vi "VisualizePXI_MultiTrig.vi"() -> ()   [LabVIEW 2018, in "Visualization.lvlib" / "VisualizeSync.lvclass"]
doc: "This VI listens for any measurement data associated with the provided PluginName and displays it to the user for analysis. The display is only suitable for data coming from the RoomAlert Plugin."
uses:
  VisualizeSync.lvclass
  <vilib>/event_ctls.llb/usereventprio.ctl
  VisualizeBase/VisualizeBase_class/Requests/clUserEventType.ctl
  <extravilib>/ChannelInstances/Tag-bool/Write With Abort.vi
  <extravilib>/ChannelInstances/Tag-bool/Read With Abort.vi
  <extravilib>/ChannelInstances/Tag-bool/Instantiate.vi
  <extravilib>/ChannelInstances/Tag-bool/EndpointRead.vi
  <vilib>/Utility/error.llb/Error Cluster From Error Code.vi
  <extravilib>/ChannelInstances/Tag-bool/Endpoint.vi
  <vilib>/ErrorRing/Error Ring.xnode
  <userlib>/NIST/NISTErrorLib/NISTErrorLib.lvlib
  VisualizeBase/VisualizeBase_class/VisualizeBase.lvclass
  <extravilib>/ChannelInstances/Tag-bool.lvlib
  TestClass/Test.lvclass
  Sync/SyncModule/SyncModule.lvlib
panel:
  in  "ModuleID":i32
  in  "Log Data":bool=TRUE
  in  "btnStop":bool
  in  "btnReset":bool
  in  "btnClearTest":bool
  out "Time Ref Offset (ns)":waveform(dbl)(graph)
  out "LockStatus":bool
  out "ErrorArray":errorcluster[](array[cluster])
  in  "PluginName":string="Sensor.RoomAlert1"
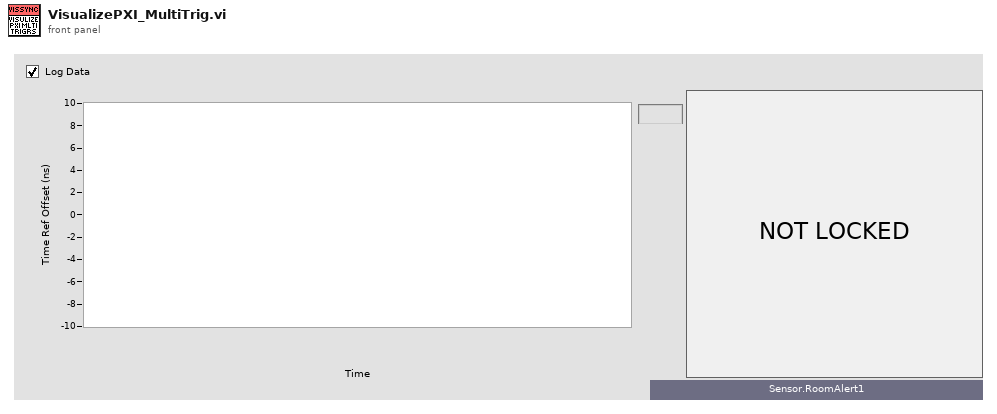
[diagram p1: front panel]
types:
  T1 = enum16{"open", "open or create", "create or replace", "create", "open (read-only)"}
  T2 = typedef "Visualization.lvlib/VisualizeBase.lvclass/clRequestEvents.ctl" = cluster{"StopRequest":refnum<user-event>, "ResetRequest":refnum<user-event>, "FP Pop In or Out":refnum<user-event>}
  T3 = typedef "SyncModule.lvlib/clBroadcastEvents.ctl" = cluster{"DidInit":refnum<user-event>, "StatusUpdate":refnum<user-event>, "ErrorReport":refnum<user-event>, "DidStop":refnum<user-event>, "PathToINI":refnum<user-event>, "TriggerTime":refnum<user-event>, "LockStatus":refnum<user-event>, "Info":refnum<user-event>, "ClockProperties":refnum<user-event>, "SyncData":refnum<user-event>}
  T4 = cluster{"seconds since 1Jan1904":timestamp, "Time Ref Offset (ns)":dbl, "Lock":bool}
  T5 = typedef "Visualization.lvlib/VisualizeBase.lvclass/clUserEventType.ctl" = cluster{"BusIndex":i8, "Data":variant}
  T6 = typedef "usereventprio.ctl" = enum32{"high priority", "normal priority"}
  T7 = typedef "Tag-bool.lvlib/))Channel.ctl" = refnum<queue>
  T8 = typedef "sizeaction.ctl" = enum32{"Minimized", "Maximized", "Resized"}
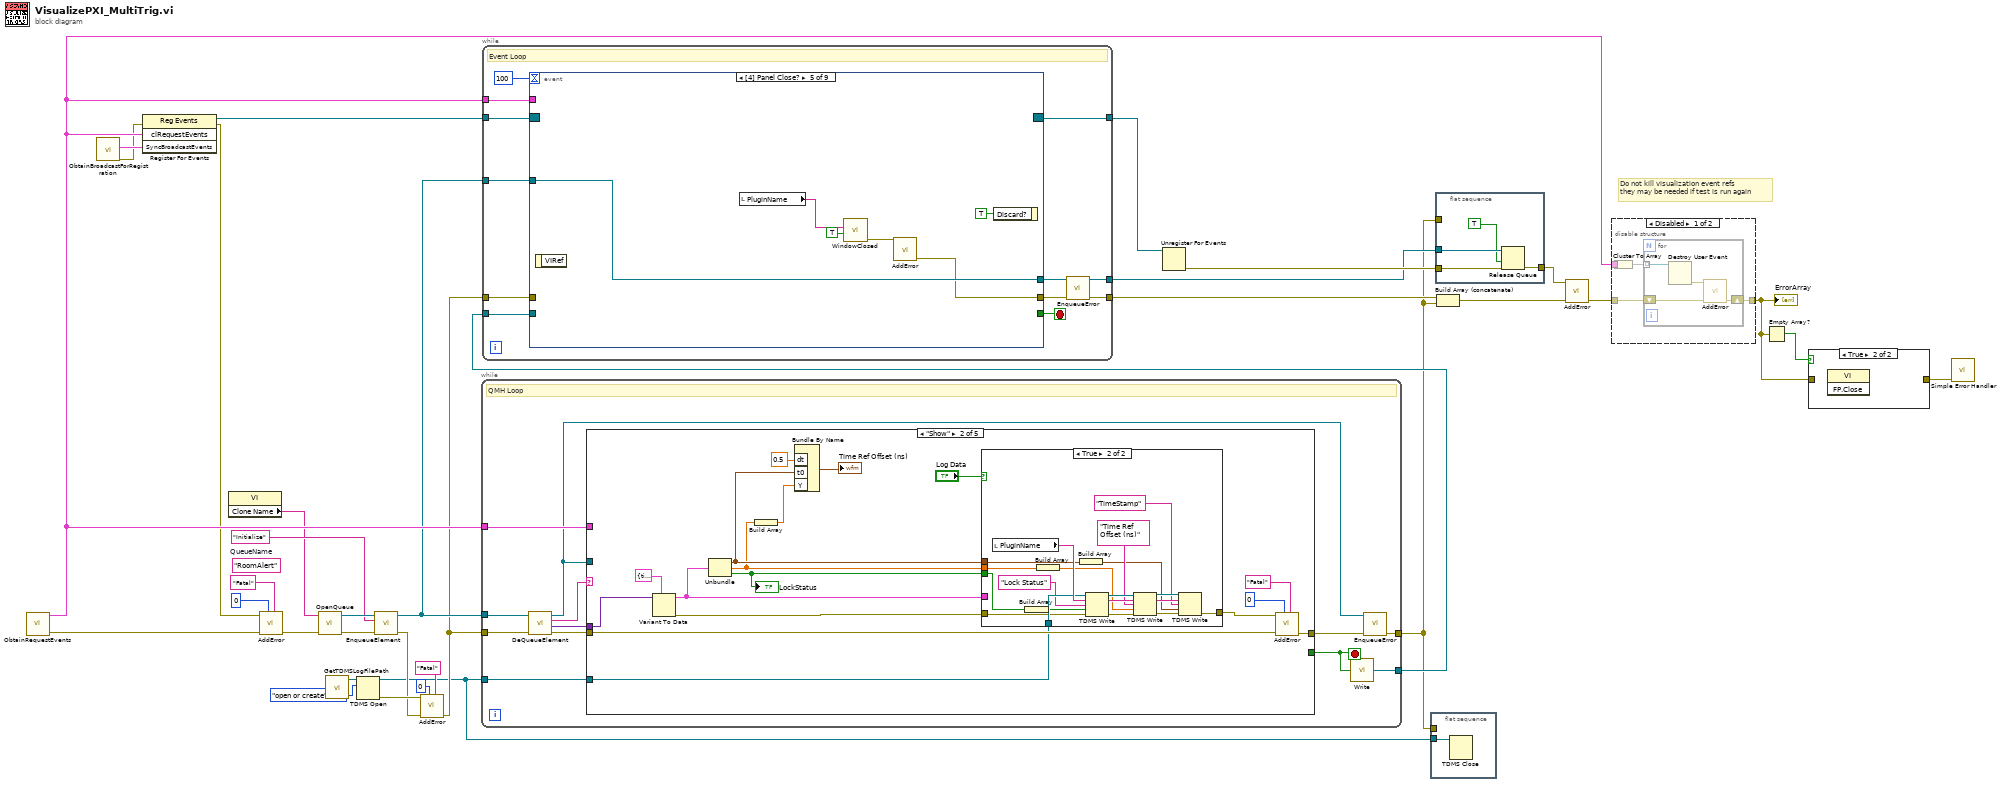
[diagram p0: block diagram]
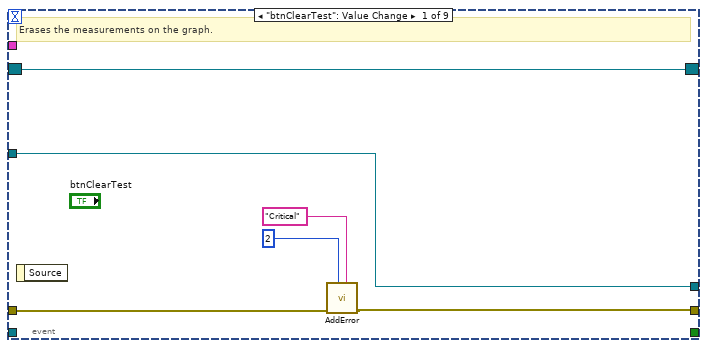
[diagram p3: hidden frame]
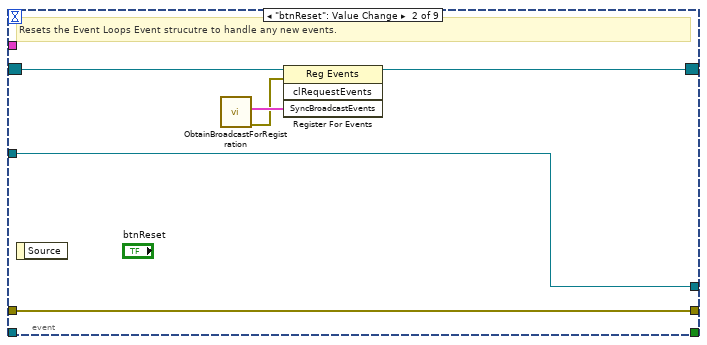
[diagram p4: hidden frame]
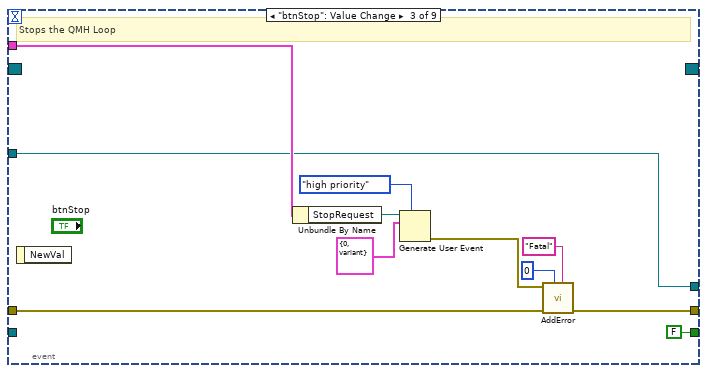
[diagram p5: hidden frame]
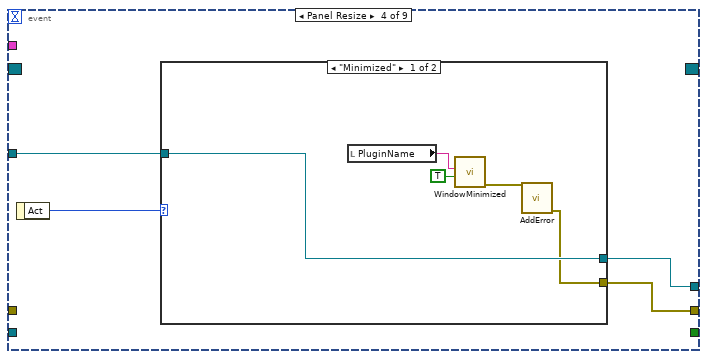
[diagram p6: hidden frame]
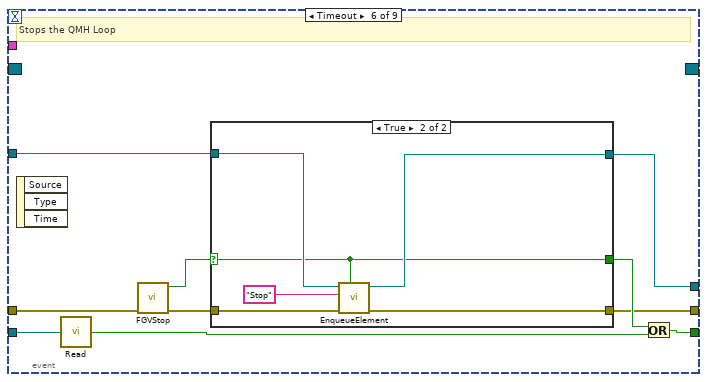
[diagram p8: hidden frame]
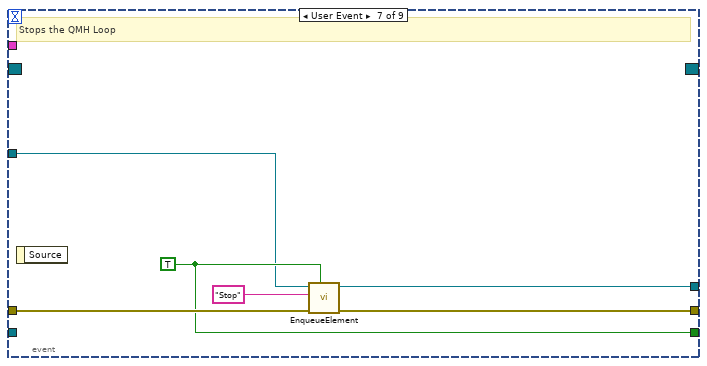
[diagram p10: hidden frame]
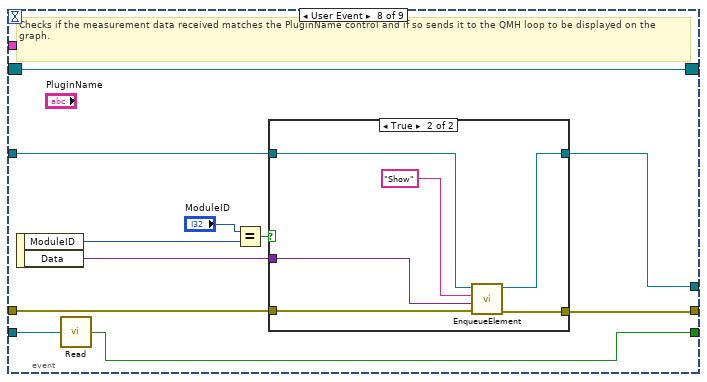
[diagram p11: hidden frame]
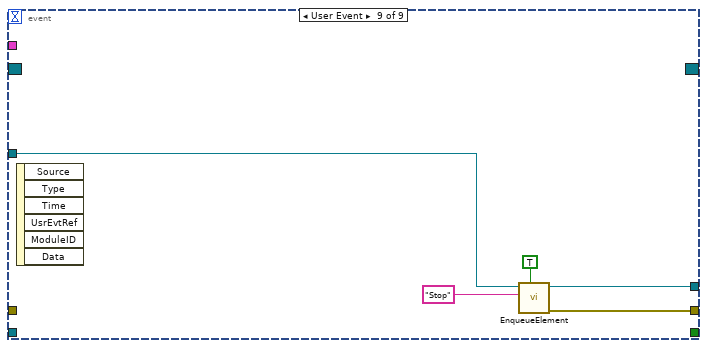
[diagram p13: hidden frame]
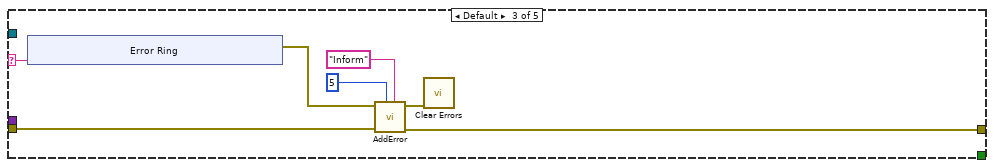
[diagram p16: hidden frame]
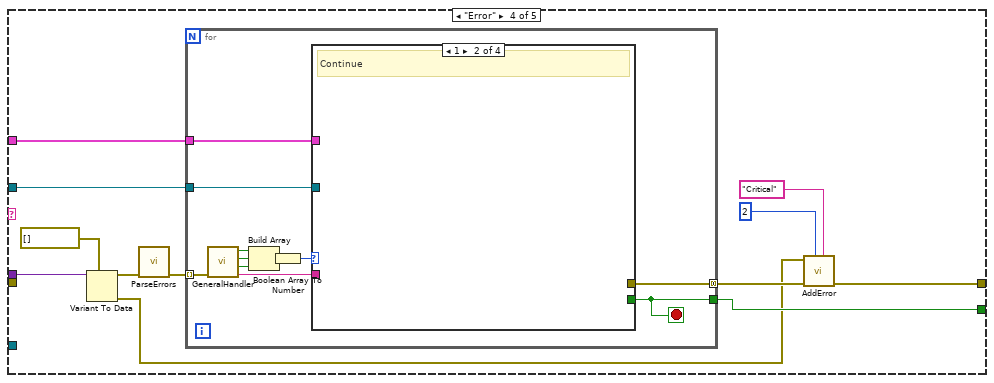
[diagram p17: hidden frame]
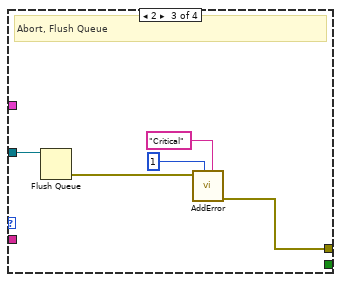
[diagram p19: hidden frame]
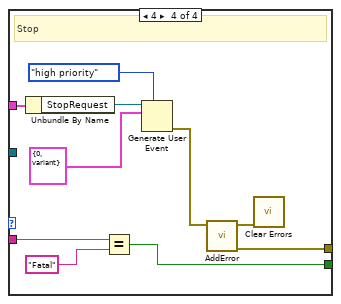
[diagram p20: hidden frame]
diagram:
  (unwired) "RoomAlert"  # QueueName
  # "Do not kill visualization event refs\nthey may be needed if test is run again"
  n1 = call "ObtainRequestEvents.vi"() -> ("Error"=w25:errorcluster[], "clRequestEvents"=w27:T2)  [unwired: 10 in]
  n2 = call "ObtainBroadcastForRegistration.vi"() -> ("error out"=w1:errorcluster, "SyncBroadcastEvents"=w2:T3)  [unwired: 10 in]
  n3 = register-events(error in=w1, w27, w2) -> (reference out=w34:refnum<event-registration>, error out=w24:errorcluster)  [unwired: 1 in]
  n4 = property class="VI"() -> ("Clone Name"=w12:string)  [unwired: 2 in, 2 out]
  n5 = call <userlib>:"AddError.vi"("Severity"="Fatal", "Priority"=u8 0, "ErrorArray In"=w25, "error in (no error)"=w24) -> ("ErrorArray Out"=w21:errorcluster[])  [unwired: 6 in, 1 out]
  n6 = call "OpenQueue.vi"("Error Array In"=w21, "QueueName"=w12) -> ("Error Array Out"=w19:errorcluster[], "queue out"=w20:refnum<queue>)  [unwired: 8 in]
  n7 = call "GetTDMSLogFilePath.vi"() -> ("TDMS Log File Path"=w11:path)  [unwired: 11 in]
  n8 = TDMS Open(10:T1."open or create" ("operation (0:open)"), 11:w11) -> (0:w8:errorcluster, 3:w4:refnum<k34>)  [unwired: 5 in]
  n9 = call "EnqueueElement.vi"("Error Array In"=w19, "Message"="Initialize", "queue in"=w20) -> ("Error Array Out"=w7:errorcluster[], "queue out"=w17:refnum<queue>)  [unwired: 7 in]
  n10 = call <userlib>:"AddError.vi"("Severity"="Fatal", "Priority"=u8 0, "ErrorArray In"=w7, "error in (no error)"=w8) -> ("ErrorArray Out"=w6:errorcluster[])  [unwired: 6 in, 1 out]
  n11 = while {
    tunnel: w6 -> [w40]
    tunnel: [w43] -> w3
    tunnel: w17 -> [w39]
    tunnel: w27 -> [w45]
    tunnel: [w36] -> w13
    tunnel: w4 -> [w35]
    stop <- w46 stop-if-true
    # "QMH Loop"
    n12 = call "DeQueueElement.vi"("Error Array In"=w40, "Queue In"=w39) -> ("Error Array Out"=w38:errorcluster[], "Data"=w41:variant, "Message"=w42:string, "Queue Out"=w37:refnum<queue>)  [unwired: 6 in]
    n13 = case shown="\"Show\"" w42 {
      selector: w42 -> [_ _ w91 _ _]
      tunnel: w41 -> [_ w60 _ w110 _]
      tunnel: w38 -> [w47 w63 w89 _ w137]
      tunnel: [w47 w64 w88 w100 w137] -> w44
      tunnel: [_ _ _ w106 TRUE] -> w46
      tunnel: w45 -> [_ _ _ w105 _]
      tunnel: w37 -> [_ _ _ w104 _]
      tunnel: w35 -> [_ w56 _ _ _]
      frame "Initialize" {
      }
      frame "Show" {
        n14 = Variant To Data(type=T4 {"seconds since 1Jan1904"=timestamp(0 s since 1904-01-01), "Time Ref Offset (ns)"=0.0, "Lock"=FALSE} ("output cluster"), Variant=w60) -> (data=w54:T4, error out=w59:errorcluster)  [unwired: 1 in]
        n15 = Unbundle(w54) -> ("seconds since 1Jan1904"=w51:timestamp, "Time Ref Offset (ns)"=w49:dbl, "Lock"=w52:bool)
        "LockStatus" <- w52
        n16 = Build Array(w49) -> (w53:dbl[])
        n17 = Bundle By Name("dt"=0.5, "t0"=w51, "Y"=w53) -> (→"Time Ref Offset (ns)":waveform(dbl))  [unwired: 1 in]
        n18 = case shown="True" "Log Data" {
          tunnel: w59 -> [w65 w82]
          tunnel: [w65 w71] -> w58
          tunnel: w56 -> [_ w83]
          tunnel: w54 -> [_ _]
          tunnel: w52 -> [_ w80]
          tunnel: w49 -> [_ w75]
          tunnel: w51 -> [_ w68]
          frame False {
          }
          frame True {
            n19 = local read "PluginName"() -> (w84:string)
            n20 = Build Array(w80) -> (w81:bool[])
            n21 = Build Array(w75) -> (w66:dbl[])
            n22 = Build Array(w68) -> (w67:timestamp[])
            n23 = TDMS Write(0:w83, 5:w84, 7:"Lock Status" ("PluginName"), 9:w81, 11:w82) -> (4:w78:refnum<k34>, 6:w77:string, 15:w76:errorcluster)  [unwired: 1 in, 1 out]
            n24 = TDMS Write(0:w78, 5:w77, 7:"Time Ref Offset (ns)" ("PluginName"), 9:w66, 11:w76) -> (4:w74:refnum<k34>, 6:w73:string, 15:w72:errorcluster)  [unwired: 1 in, 1 out]
            n25 = TDMS Write(0:w74, 5:w73, 7:"TimeStamp" ("PluginName"), 9:w67, 11:w72) -> (15:w71:errorcluster)  [unwired: 1 in, 3 out]
          }
        }
        n26 = call <userlib>:"AddError.vi"("Severity"="Fatal" ("String"), "Priority"=u8 0, "ErrorArray In"=w63, "error in (no error)"=w58) -> ("ErrorArray Out"=w64:errorcluster[])  [unwired: 6 in, 1 out]
      }
      frame Default {
        n27 = xnode "Error Ring"("parameter 0"=w91) -> ("error out"=w90:errorcluster)
        n28 = call <userlib>:"AddError.vi"("Severity"="Inform" ("String"), "Priority"=u8 5, "ErrorArray In"=w89, "error in (no error)"=w90) -> ("ErrorArray Out"=w88:errorcluster[], "error out"=w87:errorcluster)  [unwired: 6 in]
        n29 = call <vilib>:"Clear Errors.vi"("error in (no error)"=w87) -> ()  [unwired: 5 in, 2 out]
      }
      frame "Error" {
        n30 = Variant To Data(type=errorcluster[] [], Variant=w110) -> (data=w108:errorcluster[], error out=w99:errorcluster)  [unwired: 1 in]
        n31 = call <userlib>:"ParseErrors.vi"("ErrorArray"=w108) -> ("ErrorArray"=w107:errorcluster[])  [unwired: 8 in, 2 out]
        n32 = for {
          tunnel: w107 -> [w121] mode=indexing
          tunnel: [w115] -> w101 mode=concatenating
          tunnel: [w113] -> w106
          tunnel: w105 -> [w112]
          tunnel: w104 -> [w111]
          stop <- w113 stop-if-true
          n33 = call <userlib>:"GeneralHandler.vi"("error in (no error)"=w121) -> ("Severity"=w114:string, "Stop"=w118:bool, "Abort"=w119:bool, "Continue"=w120:bool)  [unwired: 6 in, 1 out]
          n34 = Build Array(w120, w119, w118) -> (w117:bool[])
          n35 = Boolean Array To Number(Boolean array=w117) -> (number=w116:u32)
          n36 = case shown="1" w116 {
            tunnel: [_ _ w126 w135] -> w115
            tunnel: w114 -> [_ _ _ w128]
            tunnel: [_ _ _ w130] -> w113
            tunnel: w112 -> [_ _ _ w129]
            tunnel: w111 -> [_ _ w122 _]
            frame 0, Default {
              # "No Dialog"
            }
            frame 1 {
              # "Continue"
            }
            frame 2 {
              # "Abort, Flush Queue"
              n37 = Flush Queue(queue=w122) -> (error out=w125:errorcluster)  [unwired: 1 in, 2 out]
              n38 = call <userlib>:"AddError.vi"("Severity"="Critical" ("String"), "Priority"=u8 1, "error in (no error)"=w125) -> ("ErrorArray Out"=w126:errorcluster[])  [unwired: 7 in, 1 out]
            }
            frame 4 {
              # "Stop"
              n39 = Unbundle By Name(w129) -> ("StopRequest"=w136:refnum<user-event>)
              n40 = Equal?(x=w128, y="Fatal" ("x")) -> (x = y?=w130:bool)
              n41 = Generate User Event(priority (normal)=usereventprio."high priority", user event=w136, event data cluster=T5 {"BusIndex"=0, "Data"=variant} ("event data")) -> (error out=w134:errorcluster)  [unwired: 1 in, 1 out]
              n42 = call <userlib>:"AddError.vi"("error in (no error)"=w134) -> ("ErrorArray Out"=w135:errorcluster[], "error out"=w131:errorcluster)  [unwired: 9 in]
              n43 = call <vilib>:"Clear Errors.vi"("error in (no error)"=w131) -> ()  [unwired: 5 in, 2 out]
            }
          }
        }
        n44 = call <userlib>:"AddError.vi"("Severity"="Critical", "Priority"=u8 2, "ErrorArray In"=w101, "error in (no error)"=w99) -> ("ErrorArray Out"=w100:errorcluster[])  [unwired: 6 in, 1 out]
      }
      frame "Stop" {
      }
    }
    n45 = call <extravilib>:"Write.vi"("element"=w46) -> ("channel"=w36:T7)  [unwired: 1 out]
    n46 = call "EnqueueError.vi"("Error Array In"=w44, "Queue in"=w37) -> ("Error Array Out"=w43:errorcluster[])  [unwired: 8 in, 1 out]
  }
  n47 = while {
    tunnel: w34 -> [w150]
    tunnel: [w144] -> w32
    tunnel: [w148] -> w33
    tunnel: w27 -> [w147]
    tunnel: w6 -> [w146]
    tunnel: w17 -> [w145]
    tunnel: [w141] -> w16
    tunnel: w13 -> [w139]
    stop <- w149 stop-if-true
    # "Event Loop"
    n48 = event shown="[4] Panel Close?" {
      selector: w150 -> [w152 w162 _ _ _ _ _ w221 _]
      dyn-events: [w152 w161 _ _ _ _ _ w221 _] -> w148
      timeout: 100 -> [_ _ _ _ _ _ _ _ _]
      tunnel: [_ _ FALSE ("Priority? (F)") _ _ w190 w211 w218 _] -> w149
      tunnel: [w153 w160 w166 w176 w184 w192 w213 w223 w236] -> w143
      tunnel: w147 -> [_ _ w165 _ _ _ _ _ _]
      tunnel: w146 -> [w154 w160 w173 _ _ w195 w214 w224 _]
      tunnel: w145 -> [w151 w159 w163 w175 w188 w194 w209 w225 w234]
      tunnel: [w151 w159 w163 w174 w188 w193 w212 w222 w235] -> w142
      tunnel: w139 -> [_ _ _ _ _ w199 _ w219 _]
      event "btnClearTest": Value Change {
        # "Erases the measurements on the graph."
        n49 = event-data() -> ()  [unwired: 1 in, 1 out]
        n50 = call <userlib>:"AddError.vi"("Severity"="Critical", "Priority"=u8 2, "ErrorArray In"=w154) -> ("ErrorArray Out"=w153:errorcluster[])  [unwired: 7 in, 1 out]
      }
      event "btnReset": Value Change {
        # "Resets the Event Loops Event strucutre to handle any new events."
        n51 = event-data() -> ()  [unwired: 1 in, 1 out]
        n52 = call "ObtainBroadcastForRegistration.vi"() -> ("error out"=w157:errorcluster, "SyncBroadcastEvents"=w158:T3)  [unwired: 10 in]
        n53 = register-events(reference=w162, error in=w157, w158) -> (reference out=w161:refnum<event-registration>)  [unwired: 1 in, 1 out]
      }
      event "btnStop": Value Change {
        # "Stops the QMH Loop"
        n54 = event-data() -> ()  [unwired: 1 in, 1 out]
        n55 = Unbundle By Name(w165) -> ("StopRequest"=w171:refnum<user-event>)
        n56 = Generate User Event(priority (normal)=usereventprio."high priority", user event=w171, event data cluster=T5 {"BusIndex"=0, "Data"=variant} ("event data")) -> (error out=w172:errorcluster)  [unwired: 1 in, 1 out]
        n57 = call <userlib>:"AddError.vi"("Severity"="Fatal" ("String"), "Priority"=u8 0, "ErrorArray In"=w173, "error in (no error)"=w172) -> ("ErrorArray Out"=w166:errorcluster[])  [unwired: 6 in, 1 out]
      }
      event Panel Resize {
        n58 = event-data() -> ("Act"=w177:T8)  [unwired: 1 in]
        n59 = case shown="\"Minimized\"" w177 {
          tunnel: [w179 _] -> w176
          tunnel: w175 -> [w180 w183]
          tunnel: [w180 w183] -> w174
          frame "Minimized" {
            n60 = local read "PluginName"() -> (w182:string)
            n61 = call "WindowMinimized.vi"("Window Minimized?"=TRUE ("Window Minimized or Clozed?"), "Module Name"=w182) -> ("error out"=w181:errorcluster)  [unwired: 9 in]
            n62 = call <userlib>:"AddError.vi"("error in (no error)"=w181) -> ("ErrorArray Out"=w179:errorcluster[])  [unwired: 9 in, 1 out]
          }
          frame "Maximized", Default {
          }
        }
      }
      event Panel Close? {
        n63 = event-data() -> ()  [unwired: 1 in, 1 out]
        n64 = local read "PluginName"() -> (w187:string)
        n65 = call "WindowClosed.vi"("Window Closed?"=TRUE ("Window Minimized or Clozed?"), "Module Name"=w187) -> ("error out"=w186:errorcluster)  [unwired: 9 in]
        n66 = call <userlib>:"AddError.vi"("error in (no error)"=w186) -> ("ErrorArray Out"=w184:errorcluster[])  [unwired: 9 in, 1 out]
        n67 = event-data("Discard?"=TRUE) -> ()  [unwired: 1 in, 1 out]
      }
      event Timeout {
        # "Stops the QMH Loop"
        n68 = event-data() -> ()  [unwired: 1 in, 3 out]
        n69 = call <extravilib>:"Read.vi"("channel"=w199) -> ("element"=w191:bool)  [unwired: 1 in, 1 out]
        n70 = call "FGVStop.vi"("Error In"=w195) -> ("Error Out"=w197:errorcluster[], "Value"=w198:bool)  [unwired: 9 in]
        n71 = case shown="True" w198 {
          selector: w198 -> [w200 w203]
          tunnel: [w202 w206] -> w192
          tunnel: w197 -> [w202 w207]
          tunnel: w194 -> [w201 w205]
          tunnel: [w201 w204] -> w193
          tunnel: [w200 w203] -> w196
          frame False {
          }
          frame True {
            n72 = call "EnqueueElement.vi"("Priority? (F)"=w203, "Error Array In"=w207, "Message"="Stop", "queue in"=w205) -> ("Error Array Out"=w206:errorcluster[], "queue out"=w204:refnum<queue>)  [unwired: 6 in]
          }
        }
        n73 = Or(x=w196, y=w191) -> (x .or. y?=w190:bool)
      }
      event User Event {
        w211 = TRUE ("Priority? (F)")
        # "Stops the QMH Loop"
        n74 = event-data() -> ()  [unwired: 1 in, 1 out]
        n75 = call "EnqueueElement.vi"("Priority? (F)"=w211, "Error Array In"=w214, "Message"="Stop", "queue in"=w209) -> ("Error Array Out"=w213:errorcluster[], "queue out"=w212:refnum<queue>)  [unwired: 6 in]
      }
      event User Event {
        # "Checks if the measurement data received matches the PluginName control and if so sends it to the QMH loop to be displayed on the graph."
        n76 = event-data() -> ("ModuleID"=w216:i32, "Data"=w217:variant)  [unwired: 1 in]
        n77 = call <extravilib>:"Read.vi"("channel"=w219) -> ("element"=w218:bool)  [unwired: 1 in, 1 out]
        n78 = Equal?(x="ModuleID", y=w216) -> (x = y?=w220:bool)
        n79 = case shown="True" w220 {
          tunnel: [w226 w232] -> w223
          tunnel: w225 -> [w227 w231]
          tunnel: w224 -> [w226 w233]
          tunnel: [w227 w230] -> w222
          tunnel: w217 -> [_ w228]
          frame False {
          }
          frame True {
            n80 = call "EnqueueElement.vi"("Error Array In"=w233, "Data"=w228, "Message"="Show", "queue in"=w231) -> ("Error Array Out"=w232:errorcluster[], "queue out"=w230:refnum<queue>)  [unwired: 6 in]
          }
        }
      }
      event User Event {
        n81 = event-data() -> ()  [unwired: 1 in, 6 out]
        n82 = call "EnqueueElement.vi"("Priority? (F)"=TRUE, "Message"="Stop", "queue in"=w234) -> ("Error Array Out"=w236:errorcluster[], "queue out"=w235:refnum<queue>)  [unwired: 7 in]
      }
    }
    n83 = call "EnqueueError.vi"("Error Array In"=w143, "Queue in"=w142) -> ("Error Array Out"=w144:errorcluster[], "Queue out"=w141:refnum<queue>)  [unwired: 8 in]
  }
  n84 = Unregister For Events(event registration refnum=w33) -> (error out=w31:errorcluster)  [unwired: 1 in]
  n85 = flat-sequence {
    tunnel: w4 -> [w239]
    tunnel: w3 -> [_]
    frame #0 {
      n86 = TDMS Close(11:w239) -> ()  [unwired: 1 in, 2 out]
    }
  }
  n87 = flat-sequence {
    tunnel: w31 -> [w243]
    tunnel: [w242] -> w29
    tunnel: w16 -> [w241]
    tunnel: w3 -> [_]
    frame #0 {
      n88 = Release Queue(queue=w241, force destroy? (F)=TRUE, error in (no error)=w243) -> (error out=w242:errorcluster)  [unwired: 2 out]
    }
  }
  n89 = Build Array (concatenate)(w32, w3) -> (w30:errorcluster[])
  n90 = call <userlib>:"AddError.vi"("ErrorArray In"=w30, "error in (no error)"=w29) -> ("ErrorArray Out"=w28:errorcluster[])  [unwired: 8 in, 1 out]
  n91 = disable-structure shown="Disabled" {
    disable-tunnel: w28 -> [w246 w252]
    disable-tunnel: w27 -> [w245 _]
    disable-tunnel: [w244 w252] -> w15
    frame Disabled {
      n92 = Cluster To Array(cluster=w245) -> (array=w247:refnum<user-event>[])
      n93 = for {
        tunnel: w247 -> [w251] mode=indexing
        shift-right: [w250] -> w244
        shift-left: w246 -> [w249]
        n94 = Destroy User Event(user event=w251) -> (error out=w248:errorcluster)  [unwired: 1 in]
        n95 = call <userlib>:"AddError.vi"("ErrorArray In"=w249, "error in (no error)"=w248) -> ("ErrorArray Out"=w250:errorcluster[])  [unwired: 8 in, 1 out]
      }
    }
    frame Enabled {
    }
  }
  "ErrorArray" <- w15
  n96 = Empty Array?(array=w15) -> (empty?=w26:bool)
  n97 = case shown="True" w26 {
    tunnel: [w253 _] -> w14
    tunnel: w15 -> [w254 _]
    frame False {
      n98 = Merge Errors(w254) -> (w253:errorcluster)
    }
    frame True {
      n99 = invoke class="VI" method="FP.Close"() -> ()  [unwired: 3 in, 3 out]
    }
  }
  n100 = call <vilib>:"Simple Error Handler.vi"("error in (no error)"=w14) -> ()  [unwired: 4 in, 5 out]
